vi "rep_cap_compose_cmd.vi"(5 "Repeated Capability":string, 7 "Attribute":T1={"Identifier"="", "Descriptive name"="", "Data Type"=enum."Integer 32", "Command"="", "Access"=2, "Range Table"="", "Read Callback"="", "Write Callback"="", "Range Callback"="", "Check Callback"="", "Rngtable Callback"="", "Coerce Callback"="", "Supported Models"="", "Instrument Options"="", "Repeated Capabilities"="", "Check Status Callback"="", "Index"=0, "Flag: OPC Wait"=FALSE, "Flag: Dont check status"=FALSE, "Flag: Cache Only"=FALSE} {"Access" items=["Read Only", "Write Only", "Read/Write"]}, 8 "error in":errorcluster, 11 "VISA resource name":refnum<visa-resource-name>) -> (0 "error out":errorcluster, 2 "Command out":string, 3 "VISA resource name out":refnum<visa-resource-name>)   [LabVIEW 2014, in "rszvl_rsidr_core.lvlib"]
uses:
  rszvl_rsidr_core.lvlib
  type_Attribute.ctl
  type_Attribute_Data_Type.ctl
  type_Error_Codes.ctl
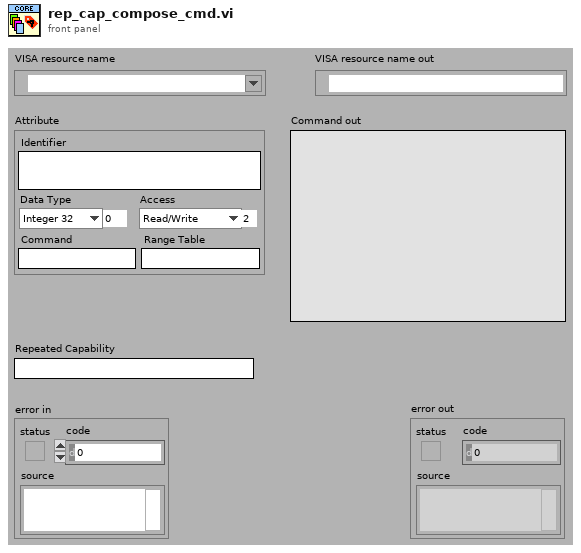
[diagram p1: front panel]
types:
  T1 = typedef "rszvl_rsidr_core.lvlib/type_Attribute.ctl" = cluster{"Identifier":string, "Descriptive name":string, "Data Type":T2, "Command":string, "Access":u16, "Range Table":string, "Read Callback":string, "Write Callback":string, "Range Callback":string, "Check Callback":string, "Rngtable Callback":string, "Coerce Callback":string, "Supported Models":string, "Instrument Options":string, "Repeated Capabilities":string, "Check Status Callback":string, "Index":i32, "Flag: OPC Wait":bool, "Flag: Dont check status":bool, "Flag: Cache Only":bool}
  T2 = typedef "rszvl_rsidr_core.lvlib/type_Attribute_Data_Type.ctl" = enum16{"Integer 32", "Double", "String", "Boolean", "None", "Integer 64"}
  T3 = typedef "rszvl_rsidr_core.lvlib/type_Error_Codes.ctl" = enum16{"No_error", "VISA_err_ResourceNotFound", "VISA_err_Timeout", "VISA_warn_MoreDataAvailable", "RS_err_MissingCallback", "RS_err_InvalidAttribute", "RS_err_InvalidValue", "RS_err_UnknownResource", "RS_err_AlreadyInitialized", "RS_err_InstrumentStatus", "RS_err_BadRepCapName", "RS_err_TypesMismatch", "RS_err_ValueNotSupported", "RS_err_InvalidRngTable", "RS_err_IDqueryFail", "RS_err_UnexpResponse", "VISA_warn_ConfigNotLoaded", "RS_err_AttributeNotReadable", "RS_err_AttributeNotWritable", "RS_err_InstrumentType", "RS_err_InstrumentOption", "VISA_err_InvalidSize", "RS_err_ReliabilityIndicator", "VISA_warn_UnknownStatus", "VISA_warn_TermCharRead", "VISA_err_IO_error"}
  T4 = enum16{"Initialize", "Get Cmd Value", "Reset Rep Cap", "Add Rep Cap", "Remove Rep Cap", "Get Rep Cap ID range", "Get Count", "Clear", "Find Name from NameID", "Get First NameID"}
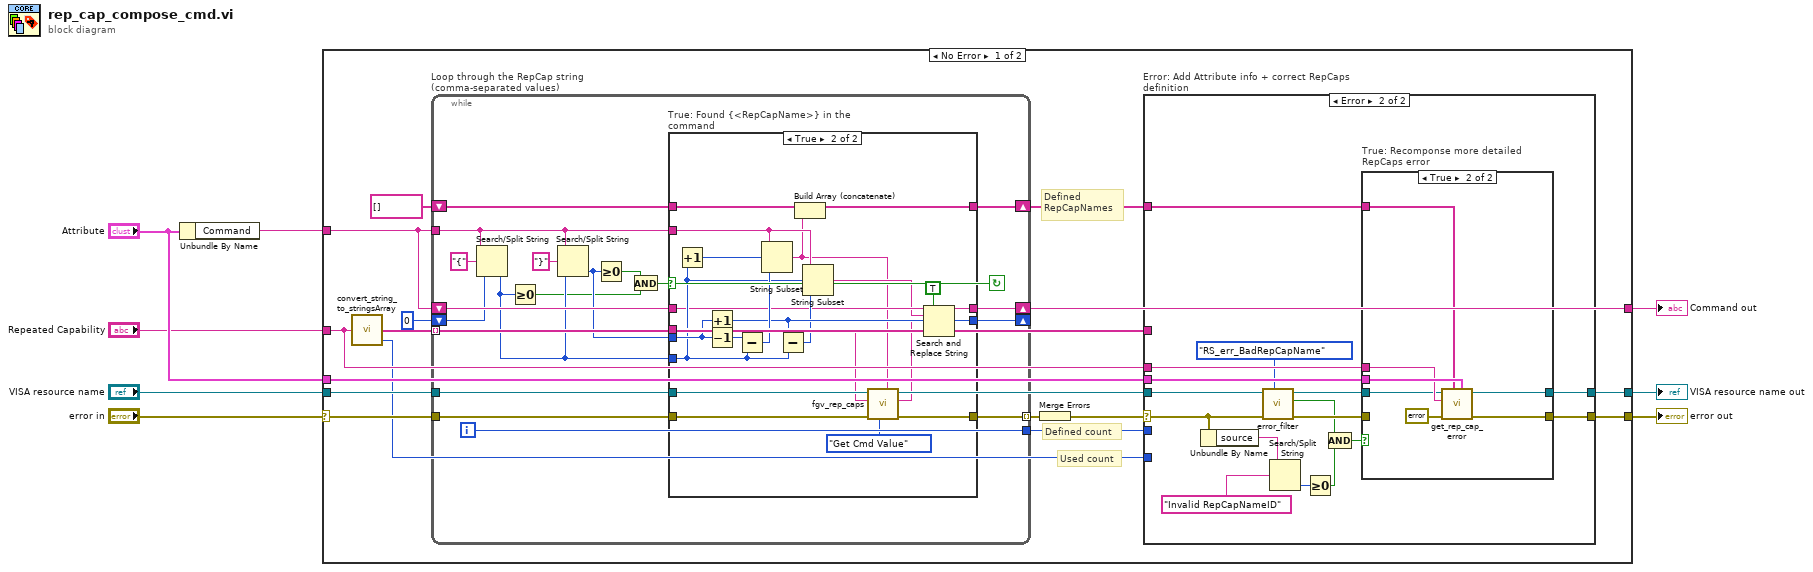
[diagram p0: block diagram]
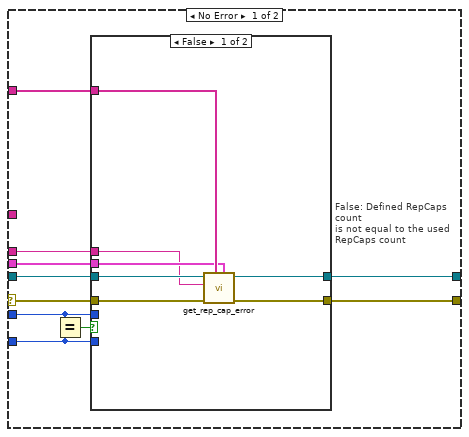
[diagram p2: hidden frame]
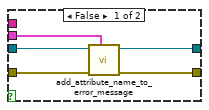
[diagram p4: hidden frame]
diagram:
  n1 = Unbundle By Name("Attribute") -> ("Command"=w1:string)
  n2 = case shown="No Error" "error in" {
    selector: "error in" -> [w23 w116]
    tunnel: "Repeated Capability" -> [w12 _]
    tunnel: [w24 w115] -> w8
    tunnel: [w19 w116] -> w7
    tunnel: w1 -> [w22 w115]
    tunnel: "VISA resource name" -> [w13 w114]
    tunnel: "Attribute" -> [w18 _]
    tunnel: [w10 w114] -> w6
    frame No Error {
      # "Defined count"
      # "Used count"
      # "Defined\nRepCapNames"
      n3 = call "convert_string_to_stringsArray.vi"("String in"=w12) -> ("string array size out"=w11:i32, "string array out"=w9:string[])  [unwired: 3 in]
      n4 = while "Loop through the RepCap string (comma-separated values)" {
        shift-right: [w89] -> w24
        shift-left: w22 -> [w88]
        tunnel: w13 -> [w86]
        tunnel: w9 -> [w85] mode=indexing
        tunnel: w22 -> [w82]
        shift-right: [w83] -> _
        shift-left: 0 -> [w72]
        tunnel: w23 -> [w87]
        tunnel: [w80] -> w15 mode=indexing
        tunnel: [w75] -> w20
        shift-right: [w73] -> w16
        shift-left: string[] [] -> [w74]
        i -> [w75]
        stop <- w71 continue-if-true
        n5 = Search/Split String(string=w82, search string/char (-)="{", offset (0)=w72) -> (offset of match=w81:i32)  [unwired: 2 out]
        n6 = Greater Or Equal To 0?(x=w81) -> (x >= 0?=w77:bool)
        n7 = Search/Split String(string=w82, search string/char (-)="}", offset (0)=w81) -> (offset of match=w78:i32)  [unwired: 2 out]
        n8 = Greater Or Equal To 0?(x=w78) -> (x >= 0?=w76:bool)
        n9 = And(x=w76, y=w77) -> (x .and. y?=w71:bool)
        n10 = case "True: Found {<RepCapName>} in the command" shown="True" w71 {
          tunnel: w88 -> [w92 w102]
          tunnel: [w92 w100] -> w89
          tunnel: [w91 w101] -> w80
          tunnel: w87 -> [w91 w112]
          tunnel: w86 -> [_ w113]
          tunnel: w85 -> [_ w111]
          tunnel: w78 -> [_ w106]
          tunnel: w81 -> [_ w103]
          tunnel: [_ w105] -> w83
          tunnel: w82 -> [_ w107]
          tunnel: w74 -> [w90 w98]
          tunnel: [w90 w97] -> w73
          frame False {
          }
          frame True {
            n11 = Increment(x=w103) -> (x+1=w110:i32)
            n12 = Increment(x=w106) -> (x+1=w105:i32)
            n13 = Decrement(x=w106) -> (x-1=w109:i32)
            n14 = Subtract(x=w109, y=w103) -> (x-y=w108:i32)
            n15 = String Subset(string=w107, offset (0)=w110, length (rest)=w108) -> (substring=w96:string)
            n16 = Subtract(x=w105, y=w103) -> (x-y=w104:i32)
            n17 = Build Array (concatenate)(w98, w96) -> (w97:string[])
            n18 = String Subset(string=w107, offset (0)=w103, length (rest)=w104) -> (substring=w99:string)
            n19 = call "fgv_rep_caps.vi"("RepCapName in (\"\")"=w96, "Operation"=T4."Get Cmd Value", "error in"=w112, "RepCapNameID in (\"\")"=w111, "VISA resource name"=w113) -> ("error out"=w101:errorcluster, "CmdValue out"=w95:string)  [unwired: 3 in, 2 out]
            n20 = Search and Replace String(replace all?=TRUE ("replace all? (F)"), input string=w102, search string=w99, replace string=w95) -> (result string=w100:string)  [unwired: 4 in, 3 out]
          }
        }
      }
      n21 = Merge Errors(w15) -> (w14:errorcluster)
      n22 = case "Error: Add Attribute info + correct RepCaps definition" shown="Error" w14 {
        selector: w14 -> [w33 w51]
        tunnel: w20 -> [w28 _]
        tunnel: [w32 w57] -> w19
        tunnel: w11 -> [w29 _]
        tunnel: w18 -> [w31 w58]
        tunnel: w12 -> [w30 w56]
        tunnel: w16 -> [w27 w44]
        tunnel: w13 -> [w26 w55]
        tunnel: [w25 w59] -> w10
        tunnel: w9 -> [_ _]
        frame No Error {
          n23 = Equal?(x=w28, y=w29) -> (x = y?=w34:bool)
          n24 = case "False: Defined RepCaps count\nis not equal to the used RepCaps count" shown="False" w34 {
            tunnel: w33 -> [w41 w43]
            tunnel: [w37 w43] -> w32
            tunnel: w31 -> [w36 _]
            tunnel: w30 -> [w35 _]
            tunnel: w29 -> [_ _]
            tunnel: w28 -> [_ _]
            tunnel: w27 -> [w39 _]
            tunnel: w26 -> [w40 w42]
            tunnel: [w38 w42] -> w25
            frame False {
              n25 = call "get_rep_cap_error.vi"("Attribute"=w36, "Defined RepCapNames in"=w39, "error in"=w41, "Repeated Capability"=w35, "VISA resource name"=w40) -> ("error out"=w37:errorcluster, "VISA resource name out"=w38:refnum<visa-resource-name>)  [unwired: 5 in]
            }
            frame True {
            }
          }
        }
        frame Error {
          n26 = Unbundle By Name(w51) -> ("source"=w45:string)
          n27 = call "error_filter.vi"("Error Enum in"=type_Error_Codes."RS_err_BadRepCapName", "error in"=w51, "VISA resource name"=w55) -> ("error out"=w52:errorcluster, "Code Detected"=w48:bool, "VISA resource name out"=w53:refnum<visa-resource-name>)  [unwired: 6 in]
          n28 = Search/Split String(string=w45, search string/char (-)="Invalid RepCapNameID") -> (offset of match=w50:i32)  [unwired: 1 in, 2 out]
          n29 = Greater Or Equal To 0?(x=w50) -> (x >= 0?=w49:bool)
          n30 = Compound Arithmetic op=AND(w48, w49) -> (w47:bool)
          n31 = case "True: Recomponse more detailed\nRepCaps error" shown="True" w47 {
            tunnel: [w63 w70] -> w59
            tunnel: w58 -> [w60 w69]
            tunnel: [w61 w68] -> w57
            tunnel: w56 -> [_ w67]
            tunnel: w53 -> [w63 w66]
            tunnel: w52 -> [w62 _]
            tunnel: w44 -> [_ w64]
            frame False {
              n32 = call "add_attribute_name_to_error_message.vi"("Attribute"=w60, "error in"=w62) -> ("error out"=w61:errorcluster)  [unwired: 8 in, 1 out]
            }
            frame True {
              n33 = call "get_rep_cap_error.vi"("Attribute"=w69, "Defined RepCapNames in"=w64, "error in"=errorcluster {"status"=FALSE, "code"=0, "source"=""}, "Repeated Capability"=w67, "VISA resource name"=w66) -> ("error out"=w68:errorcluster, "VISA resource name out"=w70:refnum<visa-resource-name>)  [unwired: 5 in]
            }
          }
        }
      }
    }
    frame Error {
    }
  }
  "error out" <- w7
  "VISA resource name out" <- w6
  "Command out" <- w8
